vi "PT 100 Temp Convert to R 1D(dbl).vi"(11 "t":dbl[](array[numeric])) -> (3 "Rt":dbl[](array[numeric]))   [LabVIEW 2012]
doc: "功能：\n\n计算温度t大于等于0，且小于等于850时的RTD电阻值。"
uses:
  PT 100 Temp Convert to R.vi
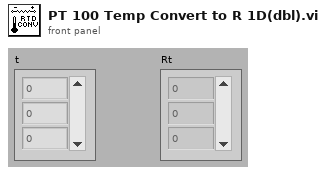
[diagram p1: front panel]
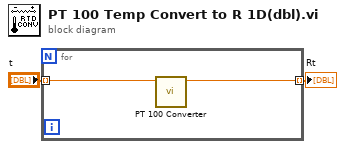
[diagram p0: block diagram]
diagram:
  n1 = for {
    tunnel: "t" -> [w4] mode=indexing
    tunnel: [w3] -> w1 mode=indexing
    n2 = call-poly "PT 100 Converter.vi"("t"=w4) -> ("Rt"=w3:dbl)  [unwired: 10 in]
  }
  "Rt" <- w1
